vi "Shutdown.vi"(8 "error in (no error)":errorcluster, 11 "AppLogger in":refnum<class "AppLogger.lvclass">) -> (0 "error out":errorcluster, 3 "AppLogger out":refnum<class "AppLogger.lvclass">)   [LabVIEW 2014, in "AppLogger.lvclass"]
uses:
  AppLogger.lvclass
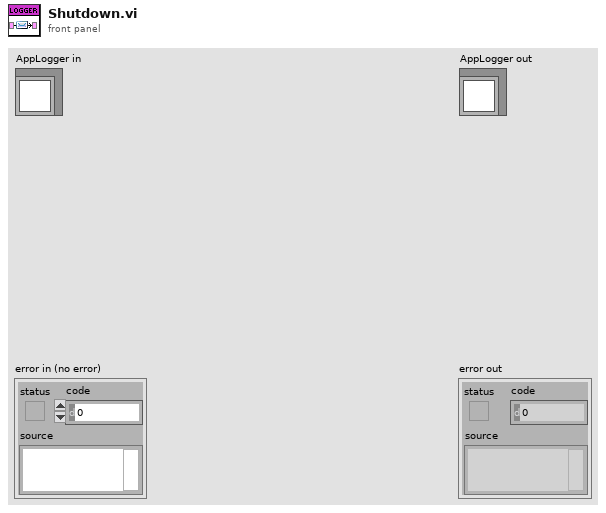
[diagram p1: front panel]
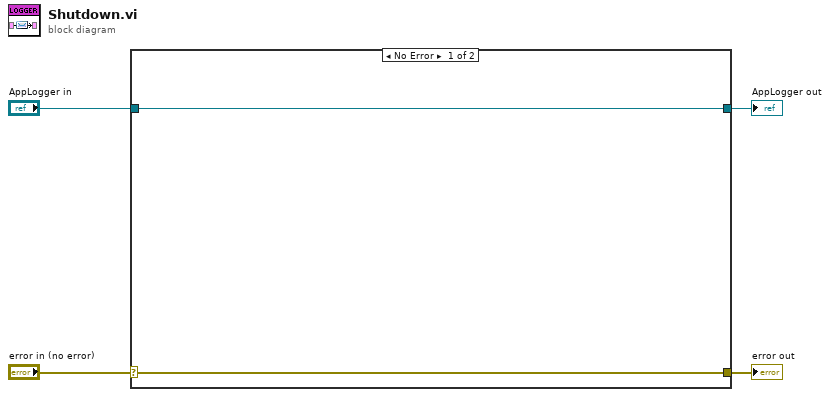
[diagram p0: block diagram]
diagram:
  n1 = case shown="No Error" "error in (no error)" {
    selector: "error in (no error)" -> [w5 w8]
    tunnel: [w5 w8] -> w3
    tunnel: [w6 w7] -> w1
    tunnel: "AppLogger in" -> [w6 w7]
    frame No Error {
    }
    frame Error {
    }
  }
  "error out" <- w3
  "AppLogger out" <- w1
